vi "Main_updated.vi"() -> ()   [LabVIEW 2016]
uses:
  Controls/Language Control.ctl
  Controls/Control_EXIT.ctl
  Controls/ctrlMainStates.ctl
  Controls/ctrlMainData.ctl
  Controls/Information_tab_type.ctl
  Controls/final data type.ctl
  <vilib>/Utility/miscctls.llb/LVPointTypeDef.ctl
  <vilib>/Utility/config.llb/Read Key (Boolean).vi
  <vilib>/Utility/config.llb/NI_LVConfig.lvlib
panel:
  in  "Exit":T1
  in  "Gas":bool
  out "Volume % Difference":dbl
  out "Progress":dbl(slide) scale=0.0..100.0
  in  "Software Version":string="1.09(US)"
  out "Sample in progress":bool
  out "Collect info done":bool
  in  "Sample method 2":u16(ring) items=["None", "Pulse Input", "Current Input", "Serial Input"]
  out "Mass % Difference":dbl
  in  "Sample \ninterval (S)":dbl=30.0
  in  "Language":T2
  in  "Collect info":bool
  in  "Export report":bool
  in  "Reset table":bool
  in  "Setpoint \n(kg/min)":dbl
  out "Data table":string[][](table)
  in  "Sample method 1":u16(ring) items=["None", "Pulse Input", "Current Input", "Serial Input"]
  in  "Begin pulse sample":bool
  in  "Transfer Data":bool
  in  "Run #":u16
  # "Flow Lifecycle Calibration Services"
  # "Mass\n(UUT)"
  # "Mass\n(Master)"
  # "Mass \n% diff"
  # "Volume\n(UUT)"
  # "Volume\n(Master)"
  # "Setpoint"
  # "Run"
  # "Select an input type"
  # "Select an input type"
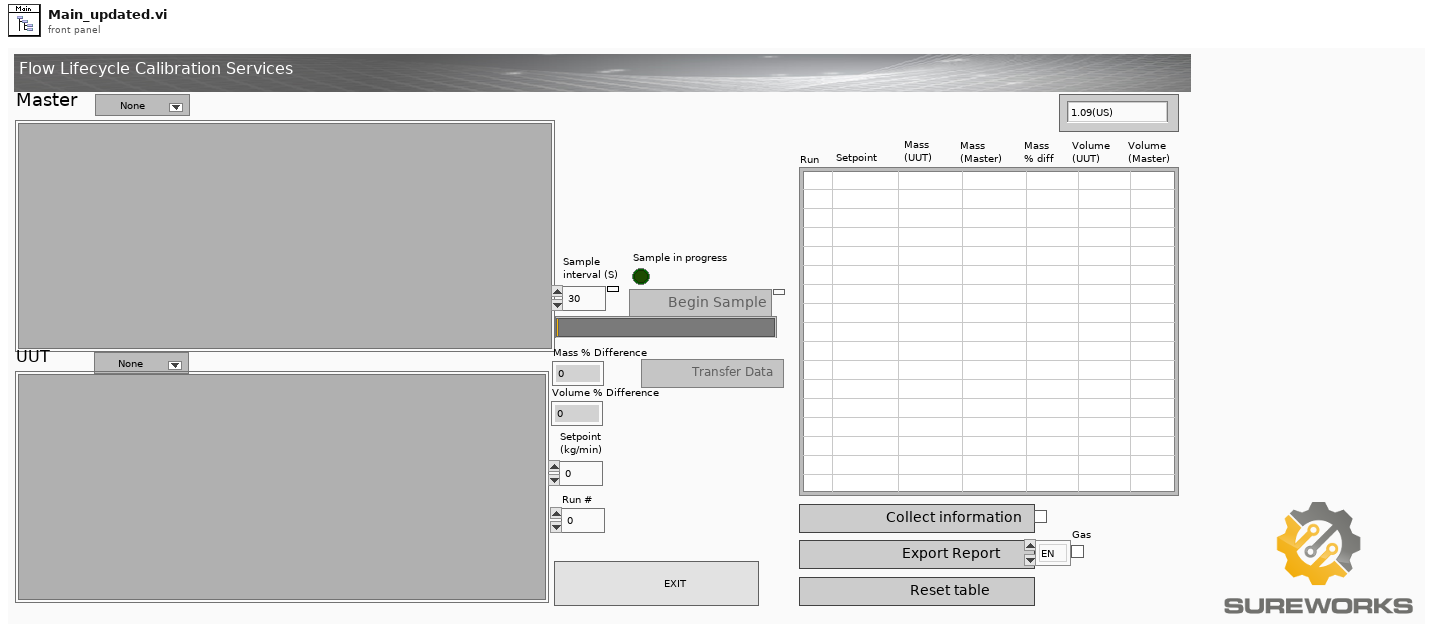
[diagram p1: front panel]
types:
  T1 = typedef "Control_EXIT.ctl" = bool
  T2 = typedef "Language Control.ctl" = enum16{"EN", "ES", "FR", "RU"}
  T3 = typedef "ctrlMainData.ctl" = cluster{"HART ports":refnum<visa-resource-name>[], "485 ports":refnum<visa-resource-name>[], "Byte order":enum16{"0-1-2-3", "2-3-0-1", "1-0-3-2", "3-2-1-0"}, "Information":T4, "Base path":path, "MasterVIRef":refnum<vi>, "UUTVIRef":refnum<vi>, "VIList":string[], "Collect info done":bool, "LeaveExcelOpen":bool, "Sample complete":bool, "Final data":T5, "StartTime":timestamp}
  T4 = typedef "Information_tab_type.ctl" = cluster{"Test Date and Time, 1":string, "Test Comments,3":string, "Sensor Serial Number,6":string, "Sensor Model,7":string, "Size,8":string, "Material,9":string, "Press rating, 10":string, "Temp rating, 11":string, "FCF, 14":string, "D1, 15":string, "D2, 16":string, "K1, 17":string, "K2, 18":string, "FD, 19":string, "Density Temp Coeff, 20":string, "Transmitter Serial Number,23":string, "Transmitter Model Number,24":string, "Mass Flow Units, 25":string, "Density Units, 26":string, "Temperature Units, 27":string, "Mass Flow Cutoff, 28":string, "Mass Flow Damping, 29":string, "Flow Direction, 30":string, "Frequency Flow Rate, 31":string, "Frequency Span, 32":string, "Flow Accuracy, 35":string, "Flow Repeatability, 36":string, "Zero Stability, 37":string, "Density Accuracy, 38":string, "Density Repeatability, 39":string, "Nomincal Flow Rate, 41":string, "Meter Zero, 43":string, "Status, 45":string, "Customer name, 46":string, "Customer address, 47":string, "Sales order number, 48":string, "Technician Name, 49":string, "ref meter, 50":string, "product code,51":string, "fluid,52":string, "fluid temp,53":string}
  T5 = typedef "final data type.ctl" = cluster{"Master final data":cluster{"Mass total":dbl, "Volume total":dbl, "Density mean":dbl}, "UUT final data":cluster{"Mass total":dbl, "Volume total":dbl, "Density mean":dbl}}
  T6 = typedef "ctrlMainStates.ctl" = enum16{"WaitforEvents", "Init", "Close", "SampleStarted", "SampleComplete", "TransferData", "UpdateSampleMethod1", "UpdateSampleMethod2", "ExportReport", "CollectInfo", "ResetTable", "BeginPulseSample"}
  T7 = enum8{"Enabled", "Disabled", "Disabled and Grayed Out"}
  T8 = typedef "LVPointTypeDef.ctl" = cluster{"Horizontal":i16, "Vertical":i16}
  T9 = cluster{"Current Path":path, "DataFiles Path":path, "ReportFiles Path":path, "SupportFiles Path":path, "ReportTemplate Path":path, "Sample_pulses_VIT_Path":path, "Sample_current_VIT_Path":path, "Sample_MODBUS_VIT_Path":path}
  T10 = typedef "NI_LVConfig.lvlib/Config Data RefNum.ctl" = refnum<k1>
  T11 = enum16{"0-1-2-3", "2-3-0-1", "1-0-3-2", "3-2-1-0"}
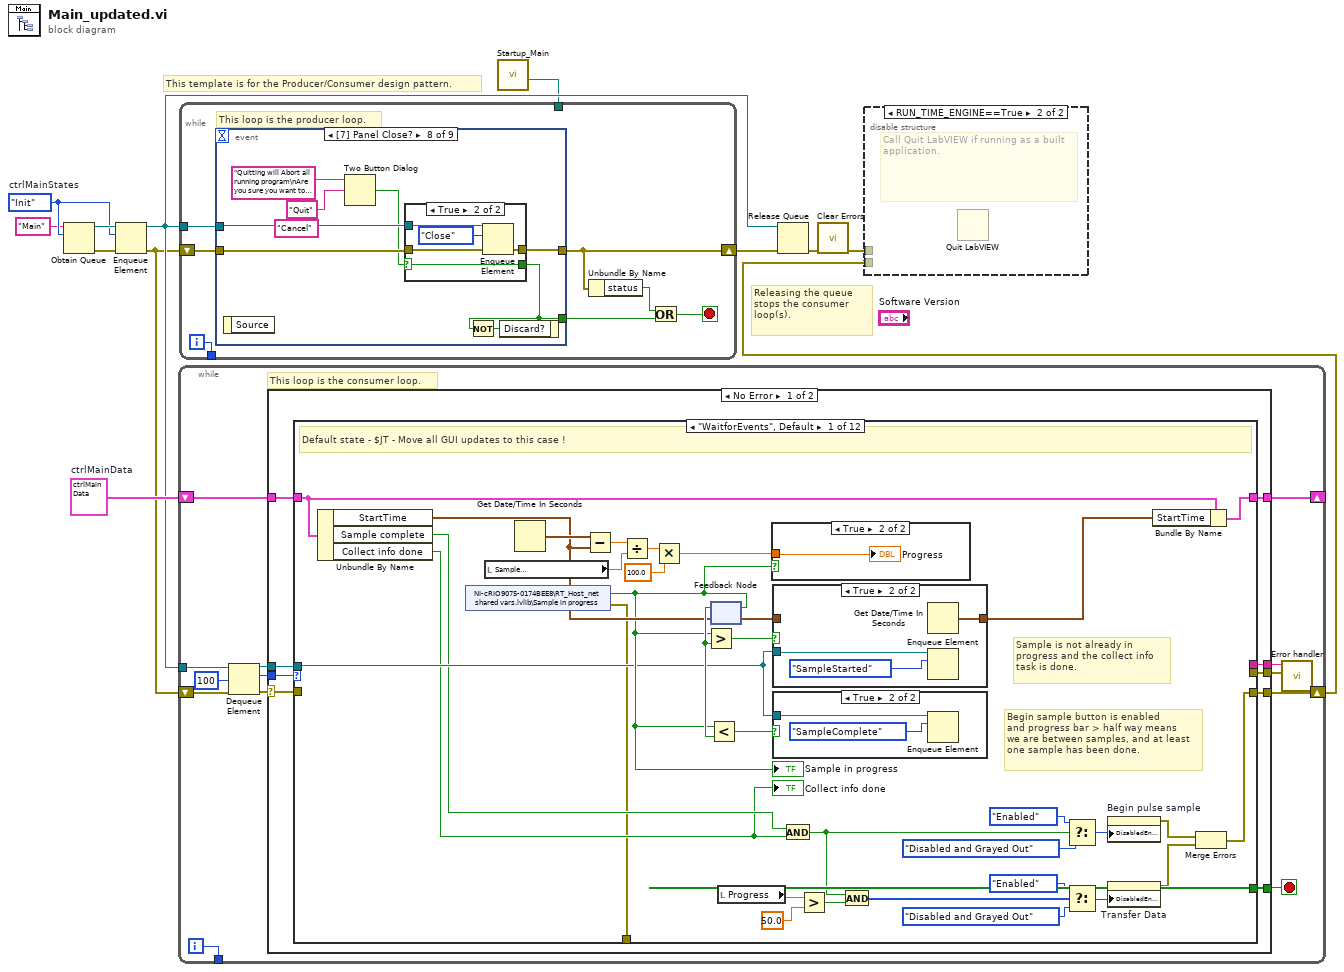
[diagram p0: block diagram]
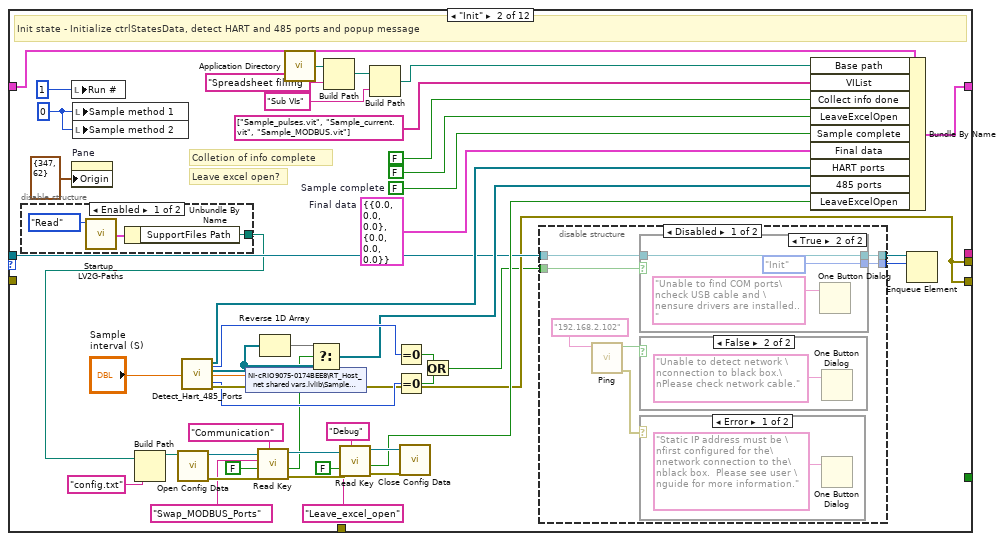
[diagram p6: hidden frame]
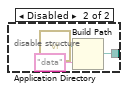
[diagram p7: hidden frame]
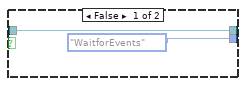
[diagram p8: hidden frame]
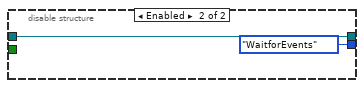
[diagram p11: hidden frame]
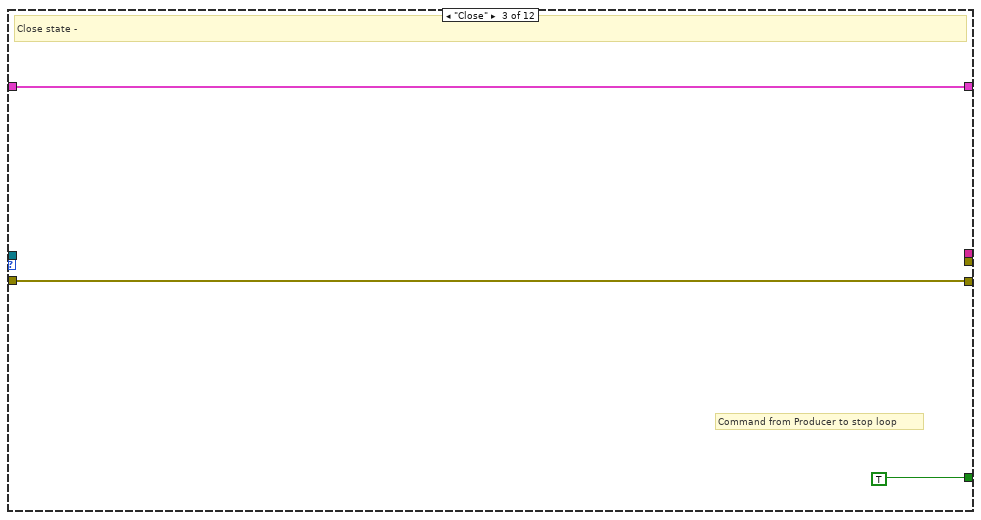
[diagram p12: hidden frame]
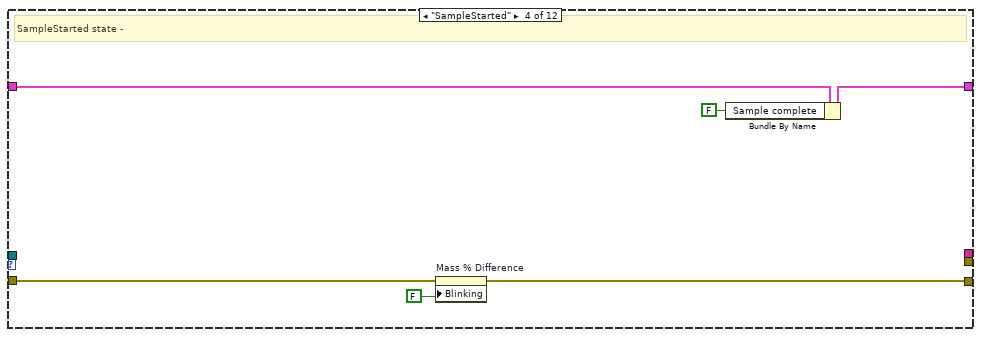
[diagram p13: hidden frame]
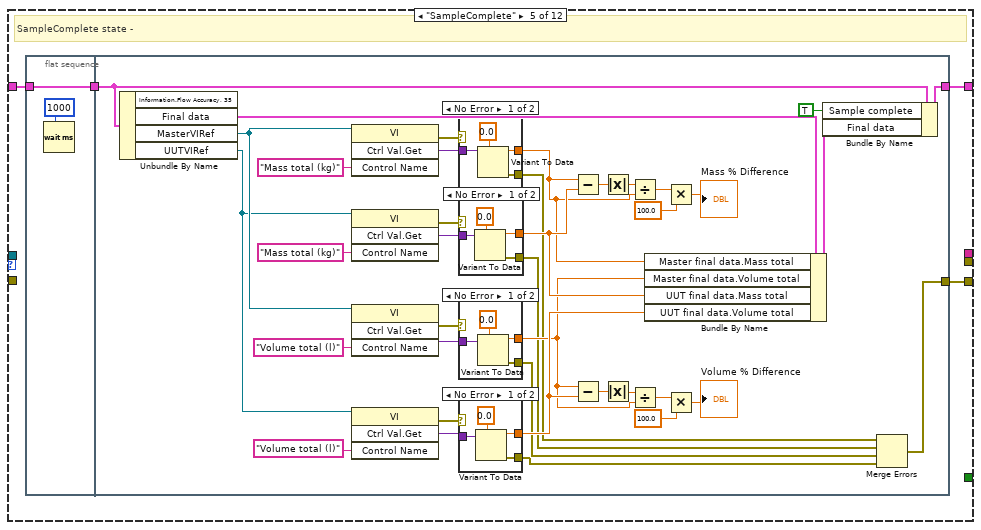
[diagram p14: hidden frame]
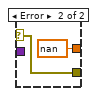
[diagram p15: hidden frame]
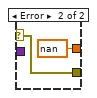
[diagram p16: hidden frame]
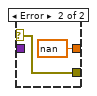
[diagram p17: hidden frame]
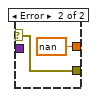
[diagram p18: hidden frame]
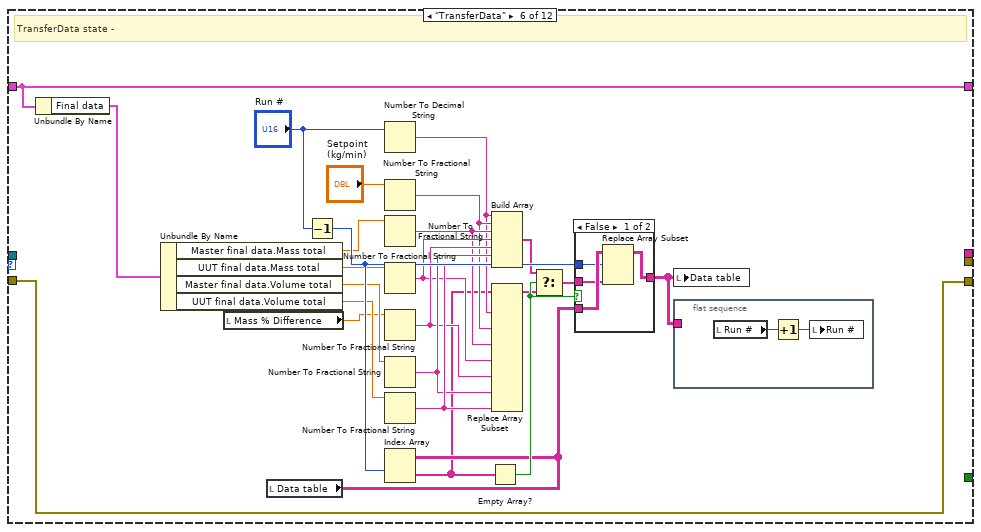
[diagram p19: hidden frame]
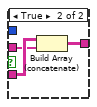
[diagram p20: hidden frame]
diagram:
  w12 = T3 {"HART ports"=[], "485 ports"=[], "Byte order"=enum."0-1-2-3", "Information"={"Test Date and Time, 1"="", "Test Comments,3"="", "Sensor Serial Number,6"="", "Sensor Model,7"="", "Size,8"="", "Material,9"="", "Press rating, 10"="", "Temp rating, 11"="", "FCF, 14"="", "D1, 15"="", "D2, 16"="", "K1, 17"="", "K2, 18"="", "FD, 19"="", "Density Temp Coeff, 20"="", "Transmitter Serial Number,23"="", "Transmitter Model Number,24"="", "Mass Flow Units, 25"="", "Density Units, 26"="", "Temperature Units, 27"="", "Mass Flow Cutoff, 28"="", "Mass Flow Damping, 29"="", "Flow Direction, 30"="", "Frequency Flow Rate, 31"="", "Frequency Span, 32"="", "Flow Accuracy, 35"="", "Flow Repeatability, 36"="", "Zero Stability, 37"="", "Density Accuracy, 38"="", "Density Repeatability, 39"="", "Nomincal Flow Rate, 41"="", "Meter Zero, 43"="", "Status, 45"="", "Customer name, 46"="", "Customer address, 47"="", "Sales order number, 48"="", "Technician Name, 49"="", "ref meter, 50"="", "product code,51"="", "fluid,52"="", "fluid temp,53"=""}, "Base path"=path "", "MasterVIRef"=refnum, "UUTVIRef"=refnum, "VIList"=[], "Collect info done"=FALSE, "LeaveExcelOpen"=FALSE, "Sample complete"=FALSE, "Final data"={"Master final data"={"Mass total"=0.0, "Volume total"=0.0, "Density mean"=0.0}, "UUT final data"={"Mass total"=0.0, "Volume total"=0.0, "Density mean"=0.0}}, "StartTime"=timestamp(0 s since 1904-01-01)}  # ctrlMainData
  w9 = ctrlMainStates."Init"  # ctrlMainStates
  # "This template is for the Producer/Consumer design pattern."
  # "Releasing the queue stops the consumer loop(s)."
  n1 = Obtain Queue(name (unnamed)="Main", element data type=w9) -> (queue out=w11:refnum<queue>, error out=w5:errorcluster)  [unwired: 3 in, 1 out]
  n2 = Enqueue Element(queue=w11, element=w9, error in (no error)=w5) -> (queue out=w10:refnum<queue>, error out=w4:errorcluster)  [unwired: 1 in, 1 out]
  n3 = while {
    tunnel: w10 -> [w25]
    shift-right: [w19] -> _
    shift-left: w12 -> [w21]
    shift-right: [w14] -> w2
    shift-left: w4 -> [w16]
    tunnel: [w13] -> _
    i -> [w13]
    stop <- w22 stop-if-true
    # "This loop is the consumer loop."
    n4 = Dequeue Element(queue=w25, timeout in ms (-1)=100, error in (no error)=w16) -> (queue out=w18:refnum<queue>, element=w23:T6, error out=w24:errorcluster)  [unwired: 1 out]
    n5 = case shown="No Error" w24 {
      selector: w24 -> [w27 w331]
      tunnel: w23 -> [w32 _]
      tunnel: [w26 TRUE] -> w22
      tunnel: w21 -> [w33 w332]
      tunnel: [w34 w332] -> w19
      tunnel: w18 -> [w31 _]
      tunnel: [w30 _] -> w15
      tunnel: [w29 _] -> w17
      tunnel: [w28 w330] -> w14
      frame No Error {
        n6 = case shown="\"WaitforEvents\", Default" w32 {
          tunnel: [w57 w109 w145 w148 w155 w222 w257 w270 w289 w310 w316 w329] -> w34
          tunnel: w33 -> [w55 w110 w145 w150 w154 w222 w255 w271 w289 w311 w318 w329]
          tunnel: w31 -> [w52 w80 _ _ _ _ _ _ _ _ _ _]
          tunnel: [_ w77 _ _ _ _ w254 w269 w285 _ _ _] -> w30
          tunnel: [_ _ _ _ _ _ _ _ "Error in PDF path.  Please check that the data output folder exists." ("Error reason") _ _ _] -> w29
          tunnel: [w36 w77 w144 w146 w152 w220 w254 w269 w285 w306 w314 w328] -> w28
          tunnel: w27 -> [_ _ w144 w147 _ w220 _ _ _ w306 w314 w328]
          tunnel: [w35 _ _ _ _ _ _ _ _ _ _ _] -> _
          tunnel: [_ _ TRUE _ _ _ _ _ _ _ _ _] -> w26
          frame "WaitforEvents", Default {
            # "Begin sample button is enabled\nand progress bar > half way means \nwe are between samples, and at least\none sample has been done."
            # "Sample is not already in\nprogress and the collect info \ntask is done."
            # "Default state - $JT - Move all GUI updates to this case !"
            n7 = Unbundle By Name(w55) -> ("StartTime"=w54:timestamp, "Sample complete"=w48:bool, "Collect info done"=w39:bool)
            "Collect info done" <- w39
            n8 = shared-variable "NI-cRIO9075-0174BEE8\\RT_Host_net shared vars.lvlib\\Sample in progress"() -> (w53:bool, error out=w35:errorcluster)  [unwired: 1 in]
            "Sample in progress" <- w53
            n9 = local read "Sample \ninterval (S)"() -> (w63:dbl)
            n10 = Get Date/Time In Seconds() -> (seconds since 1Jan1904=w61:timestamp)
            n11 = Subtract(x=w61, y=w54) -> (x-y=w62:dbl)
            n12 = Divide(x=w62, y=w63) -> (x/y=w64:dbl)
            n13 = Multiply(x=w64, y=100.0) -> (x*y=w66:dbl)
            n14 = feedback #1() -> (w59:bool)  [unwired: 1 in]
            n15 = Greater?(x=w53, y=w59) -> (0:w58:bool)
            n16 = Less?(x=w53, y=w59) -> (x < y?=w60:bool)
            n17 = feedback-in #1(w53) -> ()
            n18 = local read "Progress"() -> (w43:dbl)
            n19 = case shown="True" w53 {
              tunnel: w66 -> [_ w67]
              frame False {
              }
              frame True {
                "Progress" <- w67
              }
            }
            n20 = case shown="True" w58 {
              tunnel: w52 -> [_ w71]
              tunnel: [w70 w73] -> w56
              tunnel: w54 -> [w70 _]
              frame False {
              }
              frame True {
                n21 = Get Date/Time In Seconds() -> (seconds since 1Jan1904=w73:timestamp)
                n22 = Enqueue Element(queue=w71, element=ctrlMainStates."SampleStarted" ("ctrlStates")) -> ()  [unwired: 2 in, 3 out]
              }
            }
            n23 = case shown="True" w60 {
              tunnel: w52 -> [_ w69]
              frame False {
              }
              frame True {
                n24 = Enqueue Element(queue=w69, element=ctrlMainStates."SampleComplete" ("ctrlStates")) -> ()  [unwired: 2 in, 3 out]
              }
            }
            n25 = And(x=w48, y=w39) -> (x .and. y?=w40:bool)
            n26 = Greater?(x=w43, y=50.0) -> (0:w41:bool)
            n27 = And(x=w40, y=w41) -> (x .and. y?=w44:bool)
            n28 = Select(t=T7."Enabled" ("Disabled"), s=w40, f=T7."Disabled and Grayed Out" ("Disabled")) -> (s? t:f=w49:T7)
            n29 = Select(t=T7."Enabled" ("Disabled"), s=w44, f=T7."Disabled and Grayed Out" ("Disabled")) -> (s? t:f=w45:T7)
            n30 = property on="Begin pulse sample" class="Bool (strict)"("DisabledEnum"=w49) -> (error out=w38:errorcluster)  [unwired: 2 in, 1 out]
            n31 = property on="Transfer Data" class="Bool"("DisabledEnum"=w45) -> (error out=w37:errorcluster)  [unwired: 2 in, 1 out]
            n32 = Bundle By Name(cluster=w55, "StartTime"=w56) -> (w57:T3)
            n33 = Merge Errors(w38, w37) -> (w36:errorcluster)
          }
          frame "Init" {
            w81 = T5 {"Master final data"={"Mass total"=0.0, "Volume total"=0.0, "Density mean"=0.0}, "UUT final data"={"Mass total"=0.0, "Volume total"=0.0, "Density mean"=0.0}}  # Final data
            w82 = FALSE  # Sample complete
            w120 = u16 0 ("Run")
            # "Leave excel open?"
            # "Colletion of info complete"
            # "Init state - Initialize ctrlStatesData, detect HART and 485 ports and popup message"
            n34 = disable-structure shown="Enabled" {
              disable-tunnel: [w121 w124] -> w74
              frame Enabled {
                n35 = call "Startup_LV2G-Paths.vi"("Action"=enum16{"Read", "Write"}."Read") -> ("Paths"=w122:T9)  [unwired: 9 in, 1 out]
                n36 = Unbundle By Name(w122) -> ("SupportFiles Path"=w121:path)
              }
              frame Disabled {
                n37 = call <vilib>:"Application Directory.vi"() -> ("Application Directory"=w125:path)
                n38 = Build Path(base path=w125, name or relative path="data") -> (appended path=w124:path)
              }
            }
            n39 = local write "Run #"(u16 1 ("Run #")) -> ()
            n40 = property on="Pane" class="Pane"("Origin"=T8 {"Horizontal"=347, "Vertical"=62}) -> ()  [unwired: 2 in, 2 out]
            n41 = local write "Sample method 1"(w120) -> ()
            n42 = local write "Sample method 2"(w120) -> ()
            n43 = Build Path(base path=w74, name or relative path="config.txt") -> (appended path=w106:path)
            n44 = call <vilib>:"Open Config Data.vi"("configuration file path"=w106) -> ("error out"=w103:errorcluster, "refnum"=w104:T10)  [unwired: 8 in, 1 out]
            n45 = call "Detect_Hart_485_Ports.vi"() -> ("error out"=w118:errorcluster, "485 Ports"=w112:refnum<visa-resource-name>[], "HART ports"=w108:refnum<visa-resource-name>[], "# 485 ports found"=w114:i32, "# HART ports found"=w115:i32)  [unwired: 6 in, 1 out]
            n46 = shared-variable "NI-cRIO9075-0174BEE8\\RT_Host_net shared vars.lvlib\\Sample period"("Sample \ninterval (S)", error in=w118) -> (error out=w77:errorcluster)
            n47 = call-poly <vilib>:"Read Key.vi"("section"="Communication", "error in (no error)"=w103, "default value"=FALSE, "key"="Swap_MODBUS_Ports", "refnum"=w104) -> ("error out"=w98:errorcluster, "value"=w92:bool, "refnum out"=w99:T10)  [unwired: 3 in, 1 out]
            n48 = Reverse 1D Array(array=w112) -> (reversed array=w113:refnum<visa-resource-name>[])
            n49 = call <vilib>:"Application Directory.vi"() -> ("Application Directory"=w90:path)
            n50 = Select(t=w113, s=w92, f=w112) -> (s? t:f=w107:refnum<visa-resource-name>[])
            n51 = Build Path(base path=w90, name or relative path="Spreadsheet filling") -> (appended path=w88:path)
            n52 = call-poly <vilib>:"Read Key.vi"("section"="Debug", "error in (no error)"=w98, "default value"=FALSE, "key"="Leave_excel_open", "refnum"=w99) -> ("error out"=w97:errorcluster, "value"=w91:bool, "refnum out"=w96:T10)  [unwired: 3 in, 1 out]
            n53 = Build Path(base path=w88, name or relative path="Sub VIs") -> (appended path=w85:path)
            n54 = Equal To 0?(x=w115) -> (x = 0?=w116:bool)
            n55 = Equal To 0?(x=w114) -> (x = 0?=w117:bool)
            n56 = call <vilib>:"Close Config Data.vi"("error in (no error)"=w97, "refnum"=w96) -> ()  [unwired: 8 in, 2 out]
            n57 = Or(x=w116, y=w117) -> (x .or. y?=w76:bool)
            n58 = disable-structure shown="Disabled" {
              disable-tunnel: w80 -> [w130 w142]
              disable-tunnel: [w129 w142] -> w79
              disable-tunnel: [w128 ctrlMainStates."WaitforEvents" ("element")] -> w78
              disable-tunnel: w76 -> [w127 _]
              frame Disabled {
                n59 = call "Ping.vi"("Host IP Address"="192.168.2.102") -> ("error out"=w133:errorcluster, "success"=w132:bool)  [unwired: 8 in, 1 out]
                n60 = case shown="True" w127 {
                  tunnel: w130 -> [w135 w137]
                  tunnel: [w135 w137] -> w129
                  tunnel: [ctrlMainStates."WaitforEvents" ("element") ctrlMainStates."Init" ("element")] -> w128
                  frame False {
                  }
                  frame True {
                    n61 = One Button Dialog(message="Unable to find COM ports\ncheck USB cable and \nensure drivers are installed..") -> ()  [unwired: 1 in, 1 out]
                  }
                }
                n62 = case shown="False" w132 {
                  frame True {
                  }
                  frame False {
                    n63 = One Button Dialog(message="Unable to detect network \nconnection to black box.\nPlease check network cable.") -> ()  [unwired: 1 in, 1 out]
                  }
                }
                n64 = case shown="Error" w133 {
                  frame Error {
                    n65 = One Button Dialog(message="Static IP address must be \nfirst configured for the\nnetwork connection to the\nblack box.  Please see user \nguide for more information.") -> ()  [unwired: 1 in, 1 out]
                  }
                  frame No Error {
                  }
                }
              }
              frame Enabled {
              }
            }
            n66 = Bundle By Name(cluster=w110, "Base path"=w85, "VIList"=string[] ["Sample_pulses.vit", "Sample_current.vit", "Sample_MODBUS.vit"], "Collect info done"=FALSE, "LeaveExcelOpen"=FALSE ("Collect info done"), "Sample complete"=w82, "Final data"=w81, "HART ports"=w108, "485 ports"=w107, "LeaveExcelOpen"=w91) -> (w109:T3)
            n67 = Enqueue Element(queue=w79, element=w78) -> ()  [unwired: 2 in, 3 out]
          }
          frame "Close" {
            # "Command from Producer to stop loop"
            # "Close state -"
          }
          frame "SampleStarted" {
            # "SampleStarted state -"
            n68 = property on="Mass % Difference" class="DigNum (strict)"(error in=w147, "Blinking"=FALSE) -> (error out=w146:errorcluster)  [unwired: 1 in, 1 out]
            n69 = Bundle By Name(cluster=w150, "Sample complete"=FALSE) -> (w148:T3)
          }
          frame "SampleComplete" {
            # "SampleComplete state -"
            n70 = flat-sequence {
              tunnel: w154 -> [w157]
              tunnel: [w157] -> w153
              tunnel: [w194] -> w155
              tunnel: w153 -> [w168]
              tunnel: [w158] -> w152
              frame #0 {
                n71 = Wait (ms)(milliseconds to wait=u32 1000) -> ()  [unwired: 1 out]
              }
              frame #1 {
                n72 = Unbundle By Name(w168) -> ("Final data"=w165:T5, "MasterVIRef"=w167:refnum<vi>, "UUTVIRef"=w166:refnum<vi>)  [unwired: 1 out]
                n73 = invoke class="VI" method="Ctrl Val.Get"(reference=w167, "Control Name"="Mass total (kg)") -> (error out=w169:errorcluster, "Get Control Value Variant"=w170:variant)  [unwired: 2 in, 2 out]
                n74 = invoke class="VI" method="Ctrl Val.Get"(reference=w166, "Control Name"="Mass total (kg)") -> (error out=w172:errorcluster, "Get Control Value Variant"=w173:variant)  [unwired: 2 in, 2 out]
                n75 = invoke class="VI" method="Ctrl Val.Get"(reference=w167, "Control Name"="Volume total (l)") -> (error out=w181:errorcluster, "Get Control Value Variant"=w182:variant)  [unwired: 2 in, 2 out]
                n76 = invoke class="VI" method="Ctrl Val.Get"(reference=w166, "Control Name"="Volume total (l)") -> (error out=w184:errorcluster, "Get Control Value Variant"=w183:variant)  [unwired: 2 in, 2 out]
                n77 = case shown="No Error" w169 {
                  selector: w169 -> [_ w212]
                  tunnel: w170 -> [w211 _]
                  tunnel: [w209 nan ("Mass total")] -> w191
                  tunnel: [w208 w212] -> w162
                  frame No Error {
                    n78 = Variant To Data(type=0.0 ("Mass total"), Variant=w211) -> (data=w209:dbl, error out=w208:errorcluster)  [unwired: 1 in]
                  }
                  frame Error {
                  }
                }
                n79 = case shown="No Error" w172 {
                  selector: w172 -> [_ w218]
                  tunnel: w173 -> [w217 _]
                  tunnel: [w215 nan ("Mass total")] -> w192
                  tunnel: [w214 w218] -> w161
                  frame No Error {
                    n80 = Variant To Data(type=0.0 ("Mass total"), Variant=w217) -> (data=w215:dbl, error out=w214:errorcluster)  [unwired: 1 in]
                  }
                  frame Error {
                  }
                }
                n81 = case shown="No Error" w181 {
                  selector: w181 -> [_ w206]
                  tunnel: w182 -> [w205 _]
                  tunnel: [w203 nan ("Mass total")] -> w163
                  tunnel: [w202 w206] -> w160
                  frame No Error {
                    n82 = Variant To Data(type=0.0 ("Mass total"), Variant=w205) -> (data=w203:dbl, error out=w202:errorcluster)  [unwired: 1 in]
                  }
                  frame Error {
                  }
                }
                n83 = case shown="No Error" w184 {
                  selector: w184 -> [_ w200]
                  tunnel: w183 -> [w199 _]
                  tunnel: [w197 nan ("Mass total")] -> w193
                  tunnel: [w196 w200] -> w159
                  frame No Error {
                    n84 = Variant To Data(type=0.0 ("Mass total"), Variant=w199) -> (data=w197:dbl, error out=w196:errorcluster)  [unwired: 1 in]
                  }
                  frame Error {
                  }
                }
                n85 = Subtract(x=w191, y=w192) -> (x-y=w177:dbl)
                n86 = Subtract(x=w163, y=w193) -> (x-y=w187:dbl)
                n87 = Absolute Value(x=w177) -> (abs(x)=w178:dbl)
                n88 = Absolute Value(x=w187) -> (abs(x)=w186:dbl)
                n89 = Divide(x=w178, y=w191) -> (x/y=w175:dbl)
                n90 = Divide(x=w186, y=w163) -> (x/y=w189:dbl)
                n91 = Bundle By Name(cluster=w165, "Master final data.Mass total"=w191, "Master final data.Volume total"=w163, "UUT final data.Mass total"=w192, "UUT final data.Volume total"=w193) -> (w164:T5)
                n92 = Multiply(x=w175, y=100.0) -> (x*y=→"Mass % Difference":dbl)
                n93 = Multiply(x=w189, y=100.0) -> (x*y=→"Volume % Difference":dbl)
                n94 = Bundle By Name(cluster=w168, "Sample complete"=TRUE, "Final data"=w164) -> (w194:T3)
                n95 = Merge Errors(w162, w161, w160, w159) -> (w158:errorcluster)
              }
            }
          }
          frame "TransferData" {
            # "TransferData state -"
            n96 = Unbundle By Name(w222) -> ("Final data"=w221:T5)
            n97 = Unbundle By Name(w221) -> ("Master final data.Mass total"=w240:dbl, "UUT final data.Mass total"=w241:dbl, "Master final data.Volume total"=w242:dbl, "UUT final data.Volume total"=w243:dbl)
            n98 = local read "Mass % Difference"() -> (w236:dbl)
            n99 = local read "Data table"() -> (w231:string[][])
            n100 = Decrement(x="Run #") -> (x-1=w244:u16)
            n101 = Number To Decimal String(number="Run #") -> (decimal integer string=w225:string)  [unwired: 1 in]
            n102 = Number To Fractional String(number="Setpoint \n(kg/min)") -> (F-format string=w226:string)  [unwired: 3 in]
            n103 = Number To Fractional String(number=w240) -> (F-format string=w227:string)  [unwired: 3 in]
            n104 = Number To Fractional String(number=w241) -> (F-format string=w235:string)  [unwired: 3 in]
            n105 = Number To Fractional String(number=w236) -> (F-format string=w237:string)  [unwired: 3 in]
            n106 = Number To Fractional String(number=w242) -> (F-format string=w238:string)  [unwired: 3 in]
            n107 = Number To Fractional String(number=w243) -> (F-format string=w239:string)  [unwired: 3 in]
            n108 = Index Array(array=w231, index (row)=w244) -> (element=w224:string[])  [unwired: 1 in]
            n109 = Empty Array?(array=w224) -> (empty?=w232:bool)
            n110 = Build Array(w225, w226, w227, w235, w237, w238, w239) -> (w229:string[])
            n111 = Replace Array Subset(array=w224, new element #1=w225, new element #2=w226, new element #3=w227, new element #4=w235, new element #5=w237, new element #6=w238, new element #7=w239) -> (w228:string[])  [unwired: 7 in]
            n112 = Select(t=w229, s=w232, f=w228) -> (s? t:f=w230:string[])
            n113 = case shown="False" w232 {
              tunnel: w231 -> [w250 w253]
              tunnel: [w249 w252] -> w234
              tunnel: w244 -> [w248 _]
              tunnel: w230 -> [w247 w251]
              frame False {
                n114 = Replace Array Subset(array=w250, new element=w247, index (row)=w248) -> (w249:string[][])  [unwired: 1 in]
              }
              frame True {
                n115 = Build Array (concatenate)(w253, w251) -> (w252:string[][])
              }
            }
            n116 = local write "Data table"(w234) -> ()
            n117 = flat-sequence {
              tunnel: w234 -> [_]
              frame #0 {
                n118 = local read "Run #"() -> (w246:u16)
                n119 = Increment(x=w246) -> (x+1=w245:u16)
                n120 = local write "Run #"(w245) -> ()
              }
            }
          }
          frame "UpdateSampleMethod1" {
            # "UpdateSampleMethod1 state - UUT's sample method has changed, update the ref."
            n121 = Unbundle By Name(w255) -> ("Base path"=w259:path, "VIList"=w258:string[], "HART ports"=w261:refnum<visa-resource-name>[], "485 ports"=w260:refnum<visa-resource-name>[])  [unwired: 1 out]
            n122 = control-ref of="UUT"() -> (w263:refnum<vi>)
            n123 = Index Array(array=w261, index=1) -> (element=w265:refnum<visa-resource-name>)
            n124 = Index Array(array=w260, index=1) -> (element=w264:refnum<visa-resource-name>)
            n125 = call "Insert_subvi_to_subpanel.vi"("SubVI path"=w259, "HART resource name"=w265, "subpanel ref"=w263, "Input number"=1, "MODBUS resource name"=w264, "Index"="Sample method 1", "Array of VIs to insert"=w258) -> ("error out"=w254:errorcluster, "VI reference out"=w256:refnum<vi>)  [unwired: 3 in]
            n126 = Bundle By Name(cluster=w255, "MasterVIRef"=w256) -> (w257:T3)
          }
          frame "UpdateSampleMethod2" {
            # "UpdateSampleMethod2 state - Mater sample method has changed, update the ref."
            n127 = Unbundle By Name(w271) -> ("Base path"=w276:path, "VIList"=w275:string[], "HART ports"=w272:refnum<visa-resource-name>[], "485 ports"=w273:refnum<visa-resource-name>[])  [unwired: 1 out]
            n128 = control-ref of="Master"() -> (w277:refnum<vi>)
            n129 = Index Array(array=w273, index=0) -> (element=w279:refnum<visa-resource-name>)
            n130 = Index Array(array=w272, index=0) -> (element=w280:refnum<visa-resource-name>)
            n131 = call "Insert_subvi_to_subpanel.vi"("SubVI path"=w276, "HART resource name"=w280, "subpanel ref"=w277, "Input number"=0, "MODBUS resource name"=w279, "Index"="Sample method 2", "Array of VIs to insert"=w275) -> ("error out"=w269:errorcluster, "VI reference out"=w274:refnum<vi>)  [unwired: 3 in]
            n132 = Bundle By Name(cluster=w271, "UUTVIRef"=w274) -> (w270:T3)
          }
          frame "ExportReport" {
            # "ExportReport state -"
            n133 = Unbundle By Name(w289) -> ("Information"=w288:T4, "LeaveExcelOpen"=w287:bool)
            n134 = disable-structure shown="Enabled" {
              disable-tunnel: [w302 w305] -> w284
              frame Enabled {
                n135 = call "Startup_LV2G-Paths.vi"("Action"=enum16{"Read", "Write"}."Read") -> ("Paths"=w304:T9)  [unwired: 9 in, 1 out]
                n136 = Unbundle By Name(w304) -> ("SupportFiles Path"=w302:path)
              }
              frame Disabled {
                n137 = call <vilib>:"Application Directory.vi"() -> ("Application Directory"=w305:path)
              }
            }
            n138 = local read "Data table"() -> (w299:string[][])
            n139 = Not(x=w287) -> (.not. x?=w296:bool)
            n140 = Build Path(base path=w284, name or relative path="Test_log.csv") -> (appended path=w297:path)
            n141 = call "Build Excel File.vi"("close report? (T)"=w296, "Gas"="Gas", "Language"="Language", "Raw data"=w299, "Information"=w288) -> ("error out"=w295:errorcluster, "Excel path"=w293:path, "PDF path out"=w300:path)  [unwired: 4 in]
            n142 = Path To String(path=w293) -> (string=w291:string)
            n143 = call "writelog.vi"("PDF path in"=w300, "data file path"=w297, "Data table"=w299, "Information"=w288) -> ("error out"=w285:errorcluster)  [unwired: 7 in]
            n144 = Concatenate Strings("Error locating the Excel template:" ("Error reason"), w291) -> (w292:string)
            n145 = call "Error handler.vi"("error in"=w295, "Error reason"=w292) -> ()  [unwired: 10 in]
          }
          frame "CollectInfo" {
            # "CollectInfo state -"
            n146 = Unbundle By Name(w311) -> ("HART ports"=w313:refnum<visa-resource-name>[], "485 ports"=w312:refnum<visa-resource-name>[])
            n147 = call "Collect_Info_updated.vi"("HART ports"=w313, "485 Ports"=w312) -> ("Read Completed"=w307:bool, "Information"=w308:T4, "Byte order"=w309:T11)  [unwired: 7 in]
            n148 = Bundle By Name(cluster=w311, "Byte order"=w309, "Information"=w308, "Collect info done"=w307, "Sample complete"=w307) -> (w310:T3)
          }
          frame "ResetTable" {
            # "ResetTable state -"
            n149 = Two Button Dialog(message="Are you sure?", 2:"Yes" ("T button name (\"OK\")")) -> (T button?=w321:bool)  [unwired: 1 in]
            n150 = case shown="True" w321 {
              tunnel: w318 -> [w323 w325]
              tunnel: [w323 w325] -> w317
              tunnel: [w322 FALSE ("Collect info done")] -> w315
              frame False {
                n151 = Unbundle By Name(w323) -> ("LeaveExcelOpen"=w322:bool)
              }
              frame True {
                # "Reset table and run counter"
                # "Reset collection info status"
                n152 = local write "Run #"(u16 1 ("Run")) -> ()
                "Data table" <- string[][] [] ("Raw data")
              }
            }
            n153 = Bundle By Name(cluster=w317, "Collect info done"=w315) -> (w316:T3)
          }
          frame "BeginPulseSample" {
            # "\"BeginPulseSample\" state -"
          }
        }
      }
      frame Error {
        # "Clear errors..."
        # "Return true in any case that should stop the loop."
        n154 = call <vilib>:"Clear Errors.vi"("error in (no error)"=w331) -> ("error out"=w330:errorcluster)  [unwired: 5 in, 1 out]
      }
    }
    n155 = call "Error handler.vi"("error in"=w15, "Error reason"=w17) -> ()  [unwired: 10 in]
  }
  n156 = call "Startup_Main.vi"() -> ("path"=w1:path)  [unwired: 11 in]
  n157 = while {
    tunnel: w10 -> [w340]
    tunnel: [w339] -> _
    shift-right: [w335] -> w3
    shift-left: w4 -> [w338]
    tunnel: w1 -> [_]
    i -> [w339]
    stop <- w336 stop-if-true
    # "This loop is the producer loop."
    n158 = event shown="[7] Panel Close?" {
      selector: _ -> [_ _ _ _ _ _ _ _ _]
      dyn-events: _ -> [_ _ _ _ _ _ _ _ _]
      timeout: _ -> [_ _ _ _ _ _ _ _ _]
      tunnel: w340 -> [w344 w348 w352 w356 w360 w364 w368 w373 w388]
      tunnel: w338 -> [w342 w346 w350 w354 w358 w362 w366 w372 w387]
      tunnel: [w341 w345 w349 w353 w357 w361 w365 w371 w386] -> w335
      tunnel: [_ _ _ _ _ _ _ w369 w384] -> w334
      event "Transfer Data": Value Change {
        n159 = event-data() -> ()  [unwired: 1 in, 1 out]
        n160 = Enqueue Element(queue=w344, element=ctrlMainStates."TransferData", error in (no error)=w342) -> (error out=w341:errorcluster)  [unwired: 1 in, 2 out]
      }
      event "Sample method 1": Value Change {
        n161 = event-data() -> ()  [unwired: 1 in, 1 out]
        n162 = Enqueue Element(queue=w348, element=ctrlMainStates."UpdateSampleMethod1", error in (no error)=w346) -> (error out=w345:errorcluster)  [unwired: 1 in, 2 out]
      }
      event "Sample method 2": Value Change {
        n163 = event-data() -> ()  [unwired: 1 in, 1 out]
        n164 = Enqueue Element(queue=w352, element=ctrlMainStates."UpdateSampleMethod2", error in (no error)=w350) -> (error out=w349:errorcluster)  [unwired: 1 in, 2 out]
      }
      event "Export report": Value Change {
        n165 = event-data() -> ()  [unwired: 1 in, 1 out]
        n166 = Enqueue Element(queue=w356, element=ctrlMainStates."ExportReport", error in (no error)=w354) -> (error out=w353:errorcluster)  [unwired: 1 in, 2 out]
      }
      event "Collect info": Value Change {
        n167 = event-data() -> ()  [unwired: 1 in, 1 out]
        n168 = Enqueue Element(queue=w360, element=ctrlMainStates."CollectInfo", error in (no error)=w358) -> (error out=w357:errorcluster)  [unwired: 1 in, 2 out]
      }
      event "Reset table": Value Change {
        n169 = event-data() -> ()  [unwired: 1 in, 1 out]
        n170 = Enqueue Element(queue=w364, element=ctrlMainStates."ResetTable", error in (no error)=w362) -> (error out=w361:errorcluster)  [unwired: 1 in, 2 out]
      }
      event "Begin pulse sample": Value Change {
        n171 = event-data() -> ()  [unwired: 1 in, 1 out]
        n172 = Enqueue Element(queue=w368, element=ctrlMainStates."BeginPulseSample", error in (no error)=w366) -> (error out=w365:errorcluster)  [unwired: 1 in, 2 out]
      }
      event Panel Close? {
        (unwired) "Cancel" ("F button name (\"Cancel\")")
        n173 = event-data() -> ()  [unwired: 1 in, 1 out]
        n174 = Two Button Dialog(message="Quitting will Abort all running program\nAre you sure you want to exit?", 2:"Quit" ("T button name (\"OK\")")) -> (T button?=w370:bool)  [unwired: 1 in]
        n175 = case shown="True" w370 {
          selector: w370 -> [w377 w379]
          tunnel: w373 -> [_ w382]
          tunnel: w372 -> [w378 w381]
          tunnel: [w378 w380] -> w371
          tunnel: [w377 w379] -> w369
          frame False {
          }
          frame True {
            n176 = Enqueue Element(queue=w382, element=ctrlMainStates."Close", error in (no error)=w381) -> (error out=w380:errorcluster)  [unwired: 1 in, 2 out]
          }
        }
        n177 = Not(x=w369) -> (.not. x?=w374:bool)
        n178 = event-data("Discard?"=w374) -> ()  [unwired: 1 in, 1 out]
      }
      event Value Change {
        n179 = event-data() -> ()  [unwired: 1 in, 1 out]
        n180 = Two Button Dialog(message="Quitting will Abort all running program\nAre you sure you want to exit?", 1:"Cancel" ("F button name (\"Cancel\")"), 2:"Quit" ("T button name (\"OK\")")) -> (T button?=w385:bool)
        n181 = case shown="True" w385 {
          selector: w385 -> [w392 w394]
          tunnel: w388 -> [_ w397]
          tunnel: w387 -> [w393 w396]
          tunnel: [w393 w395] -> w386
          tunnel: [w392 w394] -> w384
          frame False {
          }
          frame True {
            n182 = Enqueue Element(queue=w397, element=ctrlMainStates."Close", error in (no error)=w396) -> (error out=w395:errorcluster)  [unwired: 1 in, 2 out]
          }
        }
      }
    }
    n183 = Unbundle By Name(w335) -> ("status"=w337:bool)
    n184 = Or(x=w337, y=w334) -> (x .or. y?=w336:bool)
  }
  n185 = Release Queue(queue=w10, error in (no error)=w3) -> (error out=w6:errorcluster)  [unwired: 1 in, 2 out]
  n186 = call <vilib>:"Clear Errors.vi"("error in (no error)"=w6) -> ("error out"=w7:errorcluster)  [unwired: 5 in, 1 out]
  n187 = disable-structure shown="RUN_TIME_ENGINE==True" {
    disable-tunnel: w7 -> [_ _]
    disable-tunnel: w2 -> [_ _]
    frame condition #0 (active) {
    }
    frame condition #1 {
      # "Call Quit LabVIEW if running as a built application."
      n188 = Quit LabVIEW() -> ()  [unwired: 1 in]
    }
  }
